vi "FlatBitArrayToMultidimentional.vi"(11 "Array in":bool[](array[boolean])) -> (3 "Array out":bool[][](array[boolean]))   [LabVIEW 2012]
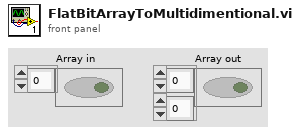
[diagram p1: front panel]
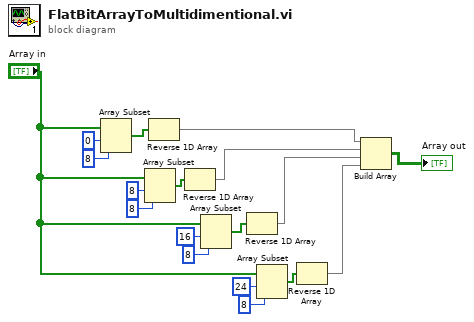
[diagram p0: block diagram]
diagram:
  n1 = Array Subset(array="Array in", index=0, length=8) -> (w11:bool[])
  n2 = Array Subset(array="Array in", index=8, length=8) -> (w12:bool[])
  n3 = Reverse 1D Array(array=w11) -> (reversed array=w14:bool[])
  n4 = Reverse 1D Array(array=w12) -> (reversed array=w15:bool[])
  n5 = Array Subset(array="Array in", index=16, length=8) -> (w13:bool[])
  n6 = Reverse 1D Array(array=w13) -> (reversed array=w16:bool[])
  n7 = Array Subset(array="Array in", index=24, length=8) -> (w18:bool[])
  n8 = Reverse 1D Array(array=w18) -> (reversed array=w17:bool[])
  n9 = Build Array(w14, w15, w16, w17) -> (→"Array out":bool[][])
